vi "VI Tree.vi"   [LabVIEW 2014, in "Associated Power Technologies 8500 Series.lvlib"]
doc: "This instrument driver supports the Associated Power Technologies 8500 Series Automated AC Power Source\".\n<B>Model Number</B> : 8505,8512,8520,8540.\n\nThe VI Tree displays all the user-callable VIs of the instrument driver in an organized table.\n\nCreated By:\nAssociated Power Technologies, Inc."
uses:
  <instrlib>/Associated Power Technologies 8500 Series/Associated Power Technologies 8500 Series.lvlib
  <instrlib>/Associated Power Technologies 8500 Series/Public/Data/Measurement/Read Voltage.vi
  <instrlib>/Associated Power Technologies 8500 Series/Public/Configure/Manual Mode/Manual Mode - Delete File.vi
  <instrlib>/Associated Power Technologies 8500 Series/Public/Configure/Manual Mode/Manual Mode - Configure THD.vi
  <instrlib>/Associated Power Technologies 8500 Series/Public/Configure/Pulse Mode/Pulse Mode - Add File.vi
  <instrlib>/Associated Power Technologies 8500 Series/Public/Configure/Step Mode/Step Mode - Edit File.vi
  <instrlib>/Associated Power Technologies 8500 Series/Public/Configure/List Mode/List Mode - Add File.vi
  <instrlib>/Associated Power Technologies 8500 Series/Public/Configure/List Mode/List Mode - Configure Fail Stop.vi
  <instrlib>/Associated Power Technologies 8500 Series/Public/Configure/List Mode/List Mode - Seq - Add Sequence.vi
  <instrlib>/Associated Power Technologies 8500 Series/Public/Configure/List Mode/List Mode - Seq - Configure THD.vi
  <instrlib>/Associated Power Technologies 8500 Series/Public/Data/Manual Mode/Manual Mode - Read THD Setting.vi
  <instrlib>/Associated Power Technologies 8500 Series/Public/Data/List Mode/List Mode - Read Editing File.vi
  <instrlib>/Associated Power Technologies 8500 Series/Public/Data/List Mode/List Mode - Seq - Read Crest Factor High Limitation Setting.vi
  <instrlib>/Associated Power Technologies 8500 Series/Public/Data/Pulse Mode/Pulse Mode - Read Editing File.vi
  <instrlib>/Associated Power Technologies 8500 Series/Public/Data/System/Read Remote IO Control Setting.vi
  <instrlib>/Associated Power Technologies 8500 Series/Public/Data/Measurement/Get Result - Index.vi
  <instrlib>/Associated Power Technologies 8500 Series/Public/Configure/Step Mode/Step Mode - Configure Trigger Source.vi
  <instrlib>/Associated Power Technologies 8500 Series/Public/Configure/System/Configure Remote IO Control.vi
  <instrlib>/Associated Power Technologies 8500 Series/Public/Data/Step Mode/Step Mode - Read Editing File.vi
  <instrlib>/Associated Power Technologies 8500 Series/Public/Configure/Pulse Mode/Pulse Mode - Configure Period.vi
panel:
  # "SEE DIAGRAM\nFOR VI Tree"
  # "Associated Power Technologies, Inc. \n28105 N Keith Drive\nLake Forest, IL 60045\n\nToll Free:  1-877-322-7693\nPhone:      1-847-367-4378\nFax:            1-847-367-4658\nEmail:        info@aptsources.com"
  # "(c) 2020 Associated Power Technologies.  ALL RIGHTS RESERVED."
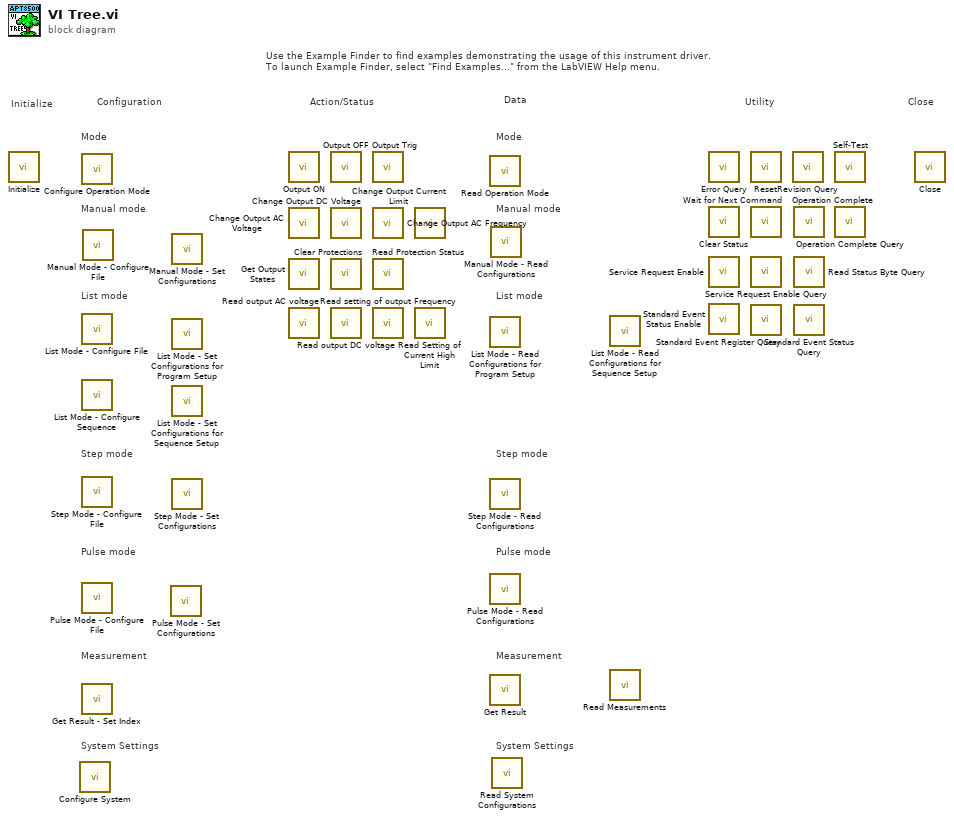
[diagram p0: block diagram]
diagram:
  # "Mode"
  # "Mode"
  # "System Settings"
  # "Measurement"
  # "Measurement"
  # "Pulse mode"
  # "Step mode"
  # "List mode"
  # "Manual mode"
  # "System Settings"
  # "Pulse mode"
  # "Step mode"
  # "List mode"
  # "Manual mode"
  # "Use the Example Finder to find examples demonstrating the usage of this instrument driver.\nTo launch Example Finder, select \"Find Examples...\" from the LabVIEW Help menu."
  # "Configuration"
  # "Utility"
  # "Data"
  # "Action/Status"
  # "Close"
  # "Initialize"
  n1 = call <instrlib>:"Initialize.vi"() -> ()  [unwired: 14 in, 2 out]
  n2 = call-poly <instrlib>:"Configure System.vi"() -> ()  [unwired: 10 in, 2 out]
  n3 = call <instrlib>:"Configure Operation Mode.vi"() -> ()  [unwired: 10 in, 2 out]
  n4 = call-poly <instrlib>:"List Mode - Configure File.vi"() -> ()  [unwired: 10 in, 2 out]
  n5 = call-poly <instrlib>:"List Mode - Configure Sequence.vi"() -> ()  [unwired: 10 in, 2 out]
  n6 = call-poly <instrlib>:"Step Mode - Configure File.vi"() -> ()  [unwired: 10 in, 2 out]
  n7 = call-poly <instrlib>:"Pulse Mode - Configure File.vi"() -> ()  [unwired: 10 in, 2 out]
  n8 = call <instrlib>:"Get Result - Set Index.vi"() -> ()  [unwired: 14 in, 2 out]
  n9 = call-poly <instrlib>:"Manual Mode - Configure File.vi"() -> ()  [unwired: 10 in, 2 out]
  n10 = call-poly <instrlib>:"Pulse Mode - Set Configurations.vi"() -> ()  [unwired: 10 in, 2 out]
  n11 = call-poly <instrlib>:"Manual Mode - Set Configurations.vi"() -> ()  [unwired: 10 in, 2 out]
  n12 = call-poly <instrlib>:"List Mode - Set Configurations for Program Setup.vi"() -> ()  [unwired: 10 in, 2 out]
  n13 = call-poly <instrlib>:"List Mode - Set Configurations for Sequence Setup.vi"() -> ()  [unwired: 10 in, 2 out]
  n14 = call-poly <instrlib>:"Step Mode - Set Configurations.vi"() -> ()  [unwired: 10 in, 2 out]
  n15 = call <instrlib>:"Output ON.vi"() -> ()  [unwired: 14 in, 2 out]
  n16 = call <instrlib>:"Change Output AC Voltage.vi"() -> ()  [unwired: 10 in, 2 out]
  n17 = call <instrlib>:"Get Output States.vi"() -> ()  [unwired: 9 in, 3 out]
  n18 = call <instrlib>:"Read output AC voltage.vi"() -> ()  [unwired: 9 in, 3 out]
  n19 = call <instrlib>:"Output OFF.vi"() -> ()  [unwired: 14 in, 2 out]
  n20 = call <instrlib>:"Change Output DC Voltage.vi"() -> ()  [unwired: 10 in, 2 out]
  n21 = call <instrlib>:"Clear Protections.vi"() -> ()  [unwired: 14 in, 2 out]
  n22 = call <instrlib>:"Read output DC voltage.vi"() -> ()  [unwired: 9 in, 3 out]
  n23 = call <instrlib>:"Output Trig.vi"() -> ()  [unwired: 14 in, 2 out]
  n24 = call <instrlib>:"Change Output AC Frequency.vi"() -> ()  [unwired: 10 in, 2 out]
  n25 = call <instrlib>:"Read Protection Status.vi"() -> ()  [unwired: 9 in, 3 out]
  n26 = call <instrlib>:"Read setting of output Frequency.vi"() -> ()  [unwired: 9 in, 3 out]
  n27 = call <instrlib>:"Change Output Current Limit.vi"() -> ()  [unwired: 10 in, 2 out]
  n28 = call <instrlib>:"Read Setting of Current High Limit.vi"() -> ()  [unwired: 9 in, 3 out]
  n29 = call <instrlib>:"Read Operation Mode.vi"() -> ()  [unwired: 9 in, 3 out]
  n30 = call-poly <instrlib>:"List Mode - Read Configurations for Program Setup.vi"() -> ()  [unwired: 9 in, 3 out]
  n31 = call-poly <instrlib>:"Step Mode - Read Configurations.vi"() -> ()  [unwired: 9 in, 3 out]
  n32 = call-poly <instrlib>:"Pulse Mode - Read Configurations.vi"() -> ()  [unwired: 9 in, 3 out]
  n33 = call-poly <instrlib>:"Get Result.vi"() -> ()  [unwired: 13 in, 3 out]
  n34 = call-poly <instrlib>:"Manual Mode - Read Configurations.vi"() -> ()  [unwired: 9 in, 3 out]
  n35 = call-poly <instrlib>:"Read System Configurations.vi"() -> ()  [unwired: 9 in, 3 out]
  n36 = call-poly <instrlib>:"List Mode - Read Configurations for Sequence Setup.vi"() -> ()  [unwired: 9 in, 3 out]
  n37 = call-poly <instrlib>:"Read Measurements.vi"() -> ()  [unwired: 13 in, 3 out]
  n38 = call <instrlib>:"Error Query.vi"() -> ()  [unwired: 12 in, 4 out]
  n39 = call <instrlib>:"Clear Status.vi"() -> ()  [unwired: 14 in, 2 out]
  n40 = call <instrlib>:"Service Request Enable.vi"() -> ()  [unwired: 14 in, 2 out]
  n41 = call <instrlib>:"Standard Event Status Enable.vi"() -> ()  [unwired: 14 in, 2 out]
  n42 = call <instrlib>:"Reset.vi"() -> ()  [unwired: 14 in, 2 out]
  n43 = call <instrlib>:"Wait for Next Command.vi"() -> ()  [unwired: 14 in, 2 out]
  n44 = call <instrlib>:"Service Request Enable Query.vi"() -> ()  [unwired: 13 in, 3 out]
  n45 = call <instrlib>:"Standard Event Register Query.vi"() -> ()  [unwired: 13 in, 3 out]
  n46 = call <instrlib>:"Revision Query.vi"() -> ()  [unwired: 11 in, 5 out]
  n47 = call <instrlib>:"Operation Complete.vi"() -> ()  [unwired: 14 in, 2 out]
  n48 = call <instrlib>:"Read Status Byte Query.vi"() -> ()  [unwired: 13 in, 3 out]
  n49 = call <instrlib>:"Standard Event Status Query.vi"() -> ()  [unwired: 13 in, 3 out]
  n50 = call <instrlib>:"Self-Test.vi"() -> ()  [unwired: 12 in, 4 out]
  n51 = call <instrlib>:"Operation Complete Query.vi"() -> ()  [unwired: 13 in, 3 out]
  n52 = call <instrlib>:"Close.vi"() -> ()  [unwired: 15 in, 1 out]
